vi "Write array of Instrument value to Ref.vi"(8 "error in (no error)":errorcluster, 10 "Array of Instruments":refnum<class "Generic Instrument.lvclass">[](array[class]), 11 "Controller in":refnum<class "Controller.lvclass">) -> (0 "error out":errorcluster, 3 "Controller out":refnum<class "Controller.lvclass">)   [LabVIEW 2014, in "Controller.lvclass"]
uses:
  Controller.lvclass
  Generic Instrument/Generic Instrument.lvclass
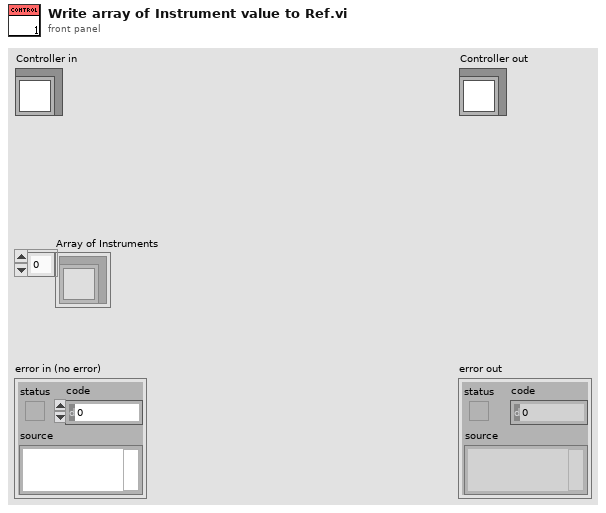
[diagram p1: front panel]
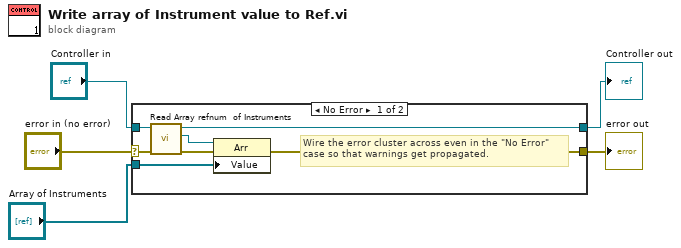
[diagram p0: block diagram]
diagram:
  n1 = case shown="No Error" "error in (no error)" {
    selector: "error in (no error)" -> [w10 w14]
    tunnel: [w8 w14] -> w4
    tunnel: [w11 w13] -> w2
    tunnel: "Controller in" -> [w12 w13]
    tunnel: "Array of Instruments" -> [w7 _]
    frame No Error {
      # "Wire the error cluster across even in the \"No Error\"\ncase so that warnings get propagated."
      n2 = call-dynamic "Read Array refnum  of Instruments.vi"("error in (no error)"=w10, "Controller in"=w12) -> ("error out"=w9:errorcluster, "Array refnum  of Instruments 2"=w6:refnum<vi>, "Controller out"=w11:refnum<class "Controller.lvclass">)  [unwired: 7 in]
      n3 = property class="Arr"(reference=w6, error in=w9, "Value"=w7) -> (error out=w8:errorcluster)  [unwired: 1 out]
    }
    frame Error {
    }
  }
  "error out" <- w4
  "Controller out" <- w2
